vi "svm_add_node_padding.vi"(8 "error in (no error)":errorcluster, 11 "Nodes":T1[](array[typedef])) -> (0 "error out":errorcluster, 3 "Padded nodes":T2[](array[typedef]))   [LabVIEW 2014]
uses:
  Controls/svm_node_padded.ctl
  Controls/svm_node.ctl
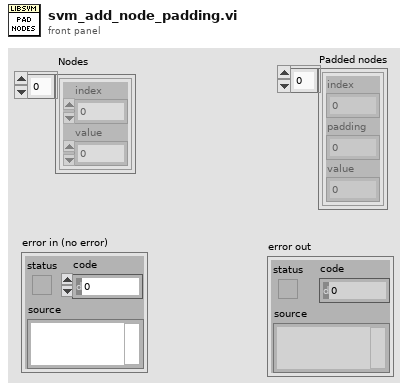
[diagram p1: front panel]
types:
  T1 = typedef "svm_node.ctl" = cluster{"index":i32, "value":dbl}
  T2 = typedef "svm_node_padded.ctl" = cluster{"index":i32, "padding":i32, "value":dbl}
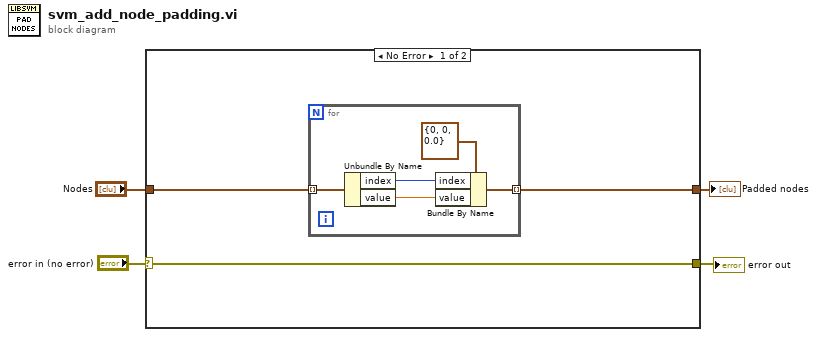
[diagram p0: block diagram]
diagram:
  n1 = case shown="No Error" "error in (no error)" {
    selector: "error in (no error)" -> [w6 w13]
    tunnel: [w6 w13] -> w4
    tunnel: [w7 _] -> w2
    tunnel: "Nodes" -> [w5 _]
    frame No Error {
      n2 = for {
        tunnel: w5 -> [w12] mode=indexing
        tunnel: [w8] -> w7 mode=indexing
        n3 = Unbundle By Name(w12) -> ("index"=w10:i32, "value"=w9:dbl)
        n4 = Bundle By Name(cluster=T2 {"index"=0, "padding"=0, "value"=0.0} ("svm_node"), "index"=w10, "value"=w9) -> (w8:T2)
      }
    }
    frame Error {
    }
  }
  "error out" <- w4
  "Padded nodes" <- w2
